vi "Camera.IMAQdx.Disconnect_LL.vi"(8 "Error In":errorcluster, 11 "Session In":T1) -> (0 "Error Out":errorcluster)   [LabVIEW 2017, in "Camera_IMAQdx.lvclass"]
uses:
  Camera_IMAQdx.lvclass
  <vilib>/userdefined/High Color/IMAQdx.ctl
  <vilib>/vision/driver/NI_Vision_Acquisition_Software.lvlib
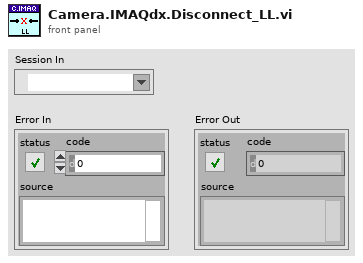
[diagram p1: front panel]
types:
  T1 = typedef "IMAQdx.ctl" = refnum<k21>
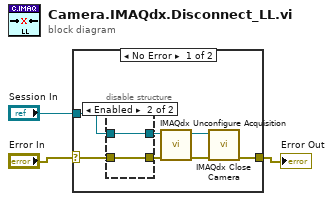
[diagram p0: block diagram]
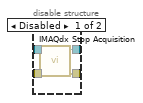
[diagram p2: hidden frame]
diagram:
  n1 = case shown="No Error" "Error In" {
    selector: "Error In" -> [w6 w17]
    tunnel: [w4 w17] -> w2
    tunnel: "Session In" -> [w5 _]
    frame No Error {
      n2 = disable-structure shown="Enabled" {
        disable-tunnel: [w14 w15] -> w10
        disable-tunnel: [w13 w16] -> w9
        disable-tunnel: w6 -> [w12 w15]
        disable-tunnel: w5 -> [w11 w16]
        frame Disabled {
          n3 = call <vilib>:"IMAQdx Stop Acquisition.vi"("error in"=w12, "Session In"=w11) -> ("error out"=w14:errorcluster, "Session Out"=w13:T1)  [unwired: 8 out]
        }
        frame Enabled {
        }
      }
      n4 = call <vilib>:"IMAQdx Unconfigure Acquisition.vi"("error in"=w10, "Session In"=w9) -> ("error out"=w7:errorcluster, "Session Out"=w8:T1)  [unwired: 8 out]
      n5 = call <vilib>:"IMAQdx Close Camera.vi"("error in"=w7, "Session In"=w8) -> ("error out"=w4:errorcluster)  [unwired: 9 out]
    }
    frame Error {
    }
  }
  "Error Out" <- w2
